vi "Add Constants Base.vi"(8 "error in (no error)":errorcluster, 10 "Value":dbl, 11 "Constant Name":string) -> (0 "error out":errorcluster)   [LabVIEW 2013]
uses:
  Constants Global.vi
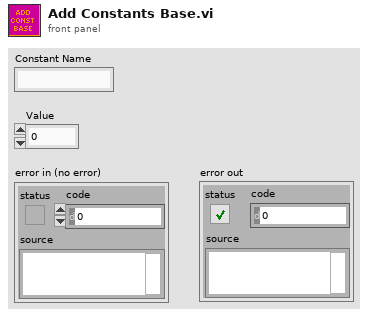
[diagram p1: front panel]
types:
  T1 = typedef "Constants Map typedef.ctl" = cluster{T2[]}[]
  T2 = typedef "Constants typedef V2.ctl" = cluster{"Constant Name":string, "Value":dbl}
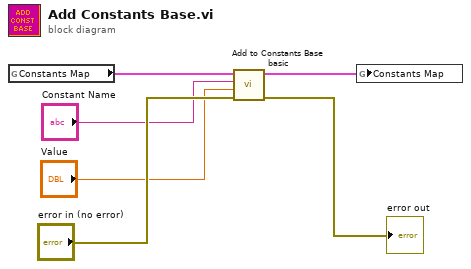
[diagram p0: block diagram]
diagram:
  n1 = global read "Constants Global.vi" "Constants Map"() -> (w3:T1)
  n2 = call "Add to Constants Base basic.vi"("error in (no error)"="error in (no error)", "Value"="Value", "Constant Name"="Constant Name", "Constants Map"=w3) -> ("Error out"=→"error out":errorcluster, "Constants Map out"=w4:T1)  [unwired: 6 in]
  n3 = global write "Constants Global.vi" "Constants Map"(w4) -> ()
